vi "AWG.vi"(1 "In":variant, 2 "Mode":u32(ring) items=["Open", "Close", "Begin", "End", "Get", "Set"]) -> (0 "Out":variant)   [LabVIEW 2014]
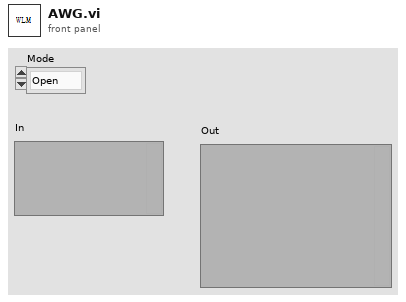
[diagram p1: front panel]
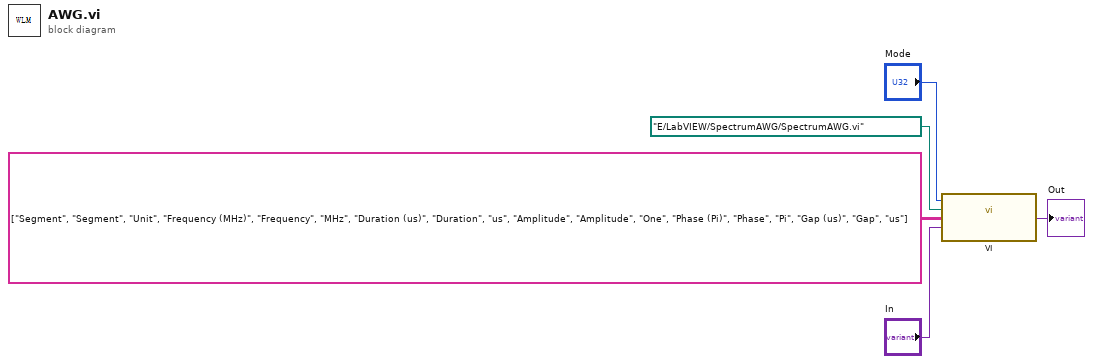
[diagram p0: block diagram]
diagram:
  n1 = call "VI.vi"("In"="In", "Names"=string[][] [["Segment", "Segment", "Unit"], ["Frequency (MHz)", "Frequency", "MHz"], ["Duration (us)", "Duration", "us"], ["Amplitude", "Amplitude", "One"], ["Phase (Pi)", "Phase", "Pi"], ["Gap (us)", "Gap", "us"]], "Path"=path "E:/LabVIEW/SpectrumAWG/SpectrumAWG.vi", "Mode"="Mode") -> ("Out"=→"Out":variant)
